vi "WriteMDF.vi"(9 "MDF In":T1 {"Latitude (waypoint)" format="%#_8g"; "Longitude  (waypoint)" format="%#_8g"}) -> ()   [LabVIEW 2010]
uses:
  6-OCU Neurons/MDF Array LatLong.ctl
  6-OCU Neurons/MDF LatLong.ctl
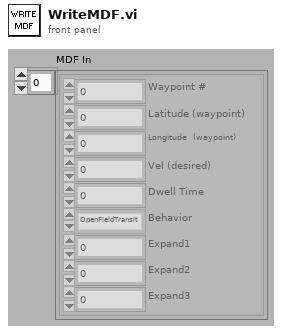
[diagram p1: front panel]
types:
  T1 = typedef "MDF Array LatLong.ctl" = T2[]
  T2 = typedef "MDF LatLong.ctl" = cluster{"Waypoint #":dbl, "Latitude (waypoint)":ext, "Longitude  (waypoint)":ext, "Vel (desired)":dbl, "Dwell Time":dbl, "Behavior":enum16{"OpenFieldTransit", "WallFollow", "LaneFollow", "ManualMode"}, "Expand1":dbl, "Expand2":dbl, "Expand3":dbl}
  T3 = enum16{"open", "replace", "create", "open or create", "replace or create", "replace or create with confirmation"}
  T4 = enum16{"OpenFieldTransit", "WallFollow", "LaneFollow", "ManualMode"}
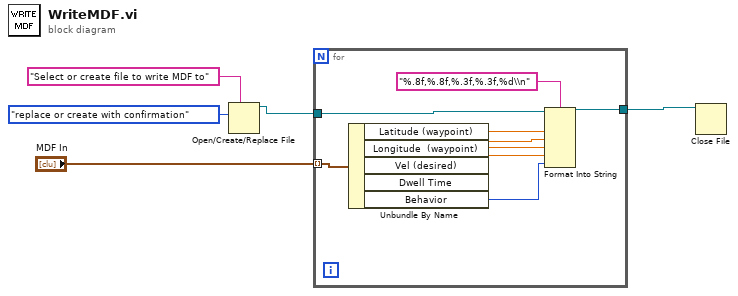
[diagram p0: block diagram]
diagram:
  n1 = Open/Create/Replace File(prompt="Select or create file to write MDF to", operation (0:open)=T3."replace or create with confirmation") -> (refnum out=w3:refnum<file>)  [unwired: 4 in, 2 out]
  n2 = for {
    tunnel: "MDF In" -> [w12] mode=indexing
    tunnel: w3 -> [w14]
    tunnel: [w13] -> w2
    n3 = Unbundle By Name(w12) -> ("Latitude (waypoint)"=w11:ext, "Longitude  (waypoint)"=w10:ext, "Vel (desired)"=w9:dbl, "Dwell Time"=w8:dbl, "Behavior"=w7:T4)
    n4 = Format Into String(format string="%.8f,%.8f,%.3f,%.3f,%d\\n", initial string=w14, w11, w10, w9, w8, w7) -> (resulting string=w13:refnum<file>)  [unwired: 1 in, 1 out]
  }
  n5 = Close File(refnum=w2) -> ()  [unwired: 1 in, 2 out]
